vi "Get Parent Folder.vi"() -> (0 "Top Level Filename":string, 1 "path":path)   [LabVIEW 2011]
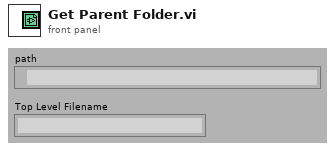
[diagram p1: front panel]
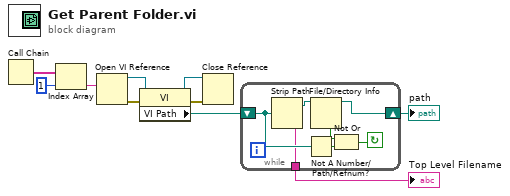
[diagram p0: block diagram]
diagram:
  n1 = Call Chain() -> (call chain=w9:string[])
  n2 = Index Array(array=w9, index=1 ("Index")) -> (element=w8:string)
  n3 = Open VI Reference(vi path=w8) -> (vi reference=w7:refnum<vi>, error out=w4:errorcluster)  [unwired: 1 in, 4 out]
  n4 = property class="VI"(reference=w7, error in=w4) -> (reference out=w5:refnum<vi>, error out=w3:errorcluster, "VI Path"=w2:path)
  n5 = Close Reference(reference=w5, error in (no error)=w3) -> ()  [unwired: 1 out]
  n6 = while {
    shift-left: w2 -> [w15]
    shift-right: [w16] -> w10
    tunnel: [w11] -> w1
    stop <- w12 continue-if-true
    n7 = Strip Path(path=w15) -> (stripped path=w17:path, name=w11:string)
    n8 = Not A Number/Path/Refnum?(number/path/refnum=w15) -> (NaN/Path/Refnum?=w13:bool)
    n9 = File/Directory Info(path=w17) -> (path out=w16:path, directory=w14:bool)  [unwired: 1 in, 5 out]
    n10 = Not Or(1:w13, 2:w14) -> (0:w12:bool)
  }
  "path" <- w10
  "Top Level Filename" <- w1
